vi "WriteScript.vi"() -> ()   [LabVIEW 2015]
uses:
  <vilib>/Utility/file.llb/Write Delimited Spreadsheet (string).vi
  Users/Sherman/Desktop/BETA_GSCS/GUI/GSP_GUI_global.vi
  <vilib>/Utility/file.llb/Read Delimited Spreadsheet (string).vi
panel:
  out "Expected Runtime":dbl
  in  "Script":string[](array[string])
  out "Gratings":T1(array[cluster])
  out "Array":T2(array[cluster])
  in  "Master Config Location":path
  in  "Littrow Config":dbl
  in  "focus sequence":bool
  in  "Clear line":bool
  out "(s)":dbl caption="Expected Runtime"
  in  "Save":bool
  in  "Line Number":dbl=1.0 min=0.0 step=1.0
  in  "Open script":bool
  in  "text file":refnum<file>
  in  "Script Name":string
  out "status":string
  in  "Add to Script Button":bool
  in  "Location of Script File":path=path "C:/GSCS Scripting/Scripts"
  in  "cluster":T3={"SI camera info"={"Observer Name"="", "object name"="", "File name base"="", "Camera Color"="Red", "Exp type tab"="", "Number of Exp"=1, "Exp time"=0.0, "CCD Readout Speed"=5, "CCD ROI Mode"=10, "Hg(Ar)"=FALSE, "Cu"=FALSE, "Ne"=FALSE, "Bulb"=FALSE, "Ar"=FALSE, "Quartz"=FALSE, "Quartz Percent"=0, "Fe"=FALSE, "Notes"="", "Target Number"="", "DomePercent"=0, "Dome"=FALSE, "Start"=0.0, "Delta"=0.0, "Steps"=0.0, "Custom Roi"={0, 4096, 1, 0, 4096, 1}}, "Configuration"={"Primary Filter"="<NO FILTER>", "Secondary Filter"="<NO FILTER>", "Slit Mask"="<NO MASK>", "Grating"="<NO GRATING>", "CS Target"=0.0, "GS Target"=0.0, "Coll Focus"=1000, "Camera Focus"=0, "Name"="", "User"="", "Date"="", "Comment"="", "use Flexure Comp?"=TRUE, "Select Mode:"=0}, "RA (HH:MM:SS.SS)"="-00:00:00.00", "DEC (HH:MM:SS.SS)"="-00:00:00.00"} {"Configuration"."Select Mode:" items=["Custom", "Imaging", "300 All", "600 UV", "600 Blue", "600 Mid", "600 Red", "1200 m0", "1200 m1", "1200 m2", "1200 m3", "1200 m4", "1200 m5", "1200 m6", "1200 m7", "1200 RESOLVE", "400 m1", "400 m2", "930 m1", "930 m2", "930 m3", "930 m4", "930 m5", "930 m6", "400WD", "930TP", "400Fermi", "400Padgett", "400Lewis", "400Crotts", "600BLee", "600RLee", "400WW", "ZZ Ceti Red", "ZZ Ceti Blue"]; "SI camera info"."DomePercent" min=0 step=1; "SI camera info"."Quartz Percent" min=0 step=1; "SI camera info"."CCD Readout Speed" items=["50 kHz, ATTN 0", "50 kHz, ATTN 2", "50 kHz, ATTN 3", "100 kHz, ATTN 0", "100 kHz, ATTN 2", "100 kHz, ATTN 3", "200 kHz, ATTN 0", "200 kHz, ATTN 2", "400 kHz, ATTN 0"]; "SI camera info"."CCD ROI Mode" items=["Imaging, 1x1  "=0, "Imaging, 2x2"=1, "Imaging, 3x3"=2, "Spectroscopic, 1x1"=3, "Spectroscopic, 2x2"=4, "Spectroscopic, 3x3"=5, "MOS, 1x1"=11, "MOS, 2x2"=12, "MOS, 3x3"=13, "Slicer"=6, "Spectroscopic, ZZ Ceti"=14, "Slit Imaging/Alignment"=7, "MOS Imaging/Alignment"=10, "Set user-defined ROI..."=21, "Custom Mode"=9]; "SI camera info"."Number of Exp" min=0 step=1; "SI camera info"."Exp time" min=0.0 format="%#.1f"}
  # "Central Wavelength (mm)"
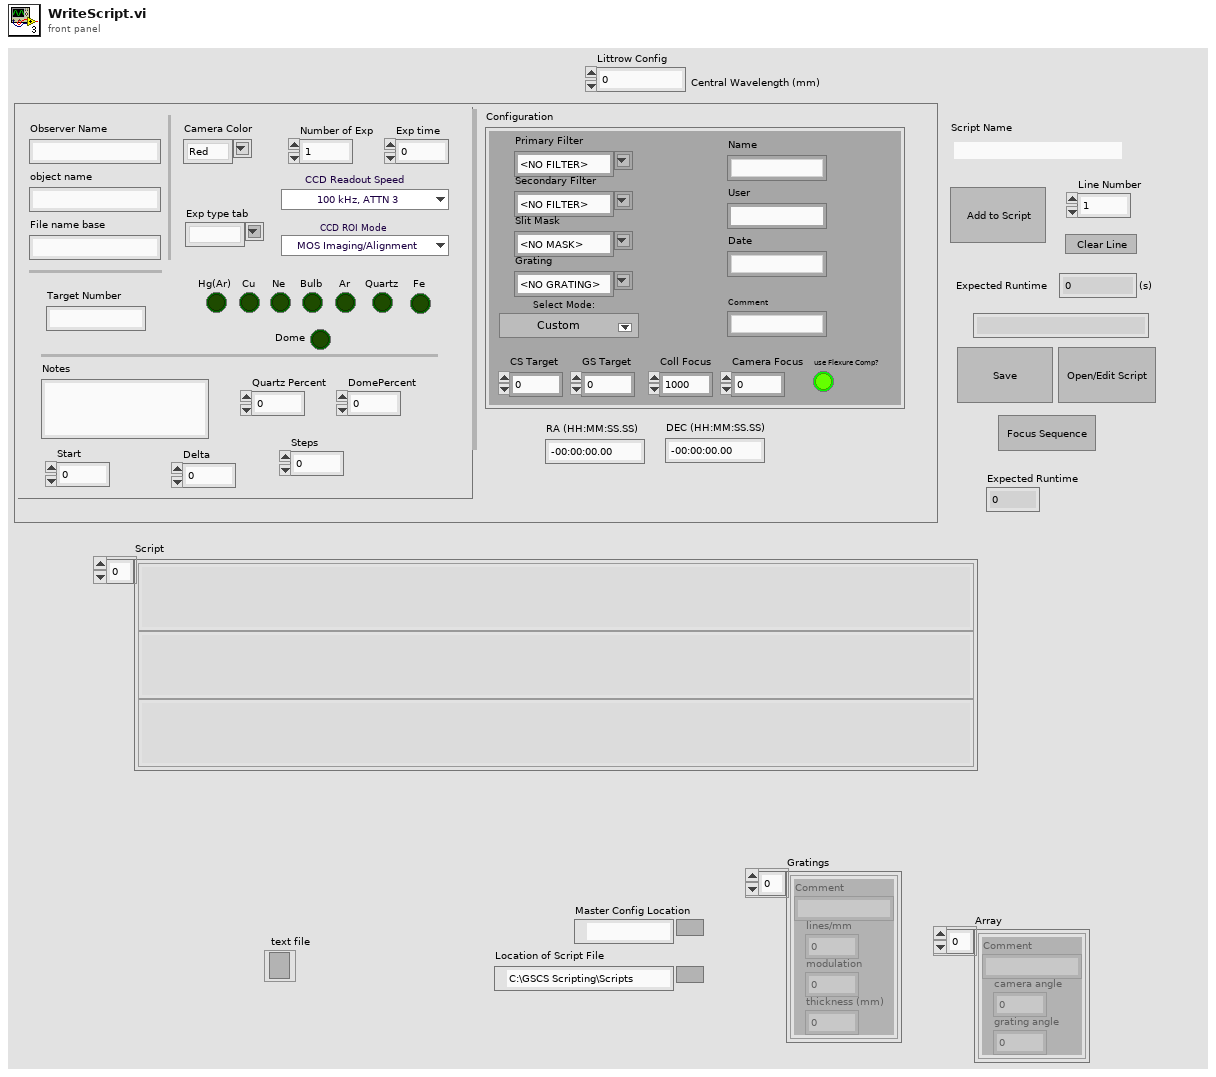
[diagram p1: front panel]
types:
  T1 = cluster{"Comment":string, "lines/mm":i32, "modulation":dbl, "thickness (mm)":dbl}[]
  T2 = cluster{"Comment":string, "camera angle":dbl, "grating angle":dbl}[]
  T3 = cluster{"SI camera info":cluster{"Observer Name":string, "object name":string, "File name base":string, "Camera Color":string, "Exp type tab":string, "Number of Exp":i32, "Exp time":dbl, "CCD Readout Speed":u8, "CCD ROI Mode":u16, "Hg(Ar)":bool, "Cu":bool, "Ne":bool, "Bulb":bool, "Ar":bool, "Quartz":bool, "Quartz Percent":i32, "Fe":bool, "Notes":string, "Target Number":string, "DomePercent":i32, "Dome":bool, "Start":dbl, "Delta":dbl, "Steps":dbl, "Custom Roi":cluster{i32, i32, i32, i32, i32, i32}}, "Configuration":cluster{"Primary Filter":string, "Secondary Filter":string, "Slit Mask":string, "Grating":string, "CS Target":dbl, "GS Target":dbl, "Coll Focus":i32, "Camera Focus":i32, "Name":string, "User":string, "Date":string, "Comment":string, "use Flexure Comp?":bool, "Select Mode:":u16}, "RA (HH:MM:SS.SS)":string, "DEC (HH:MM:SS.SS)":string}
  T4 = cluster{"Comment":string, "lines/mm":i32, "modulation":dbl, "thickness (mm)":dbl}
  T5 = cluster{"Serial Origin":i32, "Serial Length":i32, "Serial Binning":i32, "Parallel Origin":i32, "Parallel Length":i32, "Parallel Binning":i32}
  T6 = cluster{"Primary Filter Names":string[], "Secondary Filter Names":string[], "Grating Names":string[], "Slit Mask Names":string[], "Standard Observing Modes":string[]}
  T7 = cluster{"Comment":string, "camera angle":dbl, "grating angle":dbl}
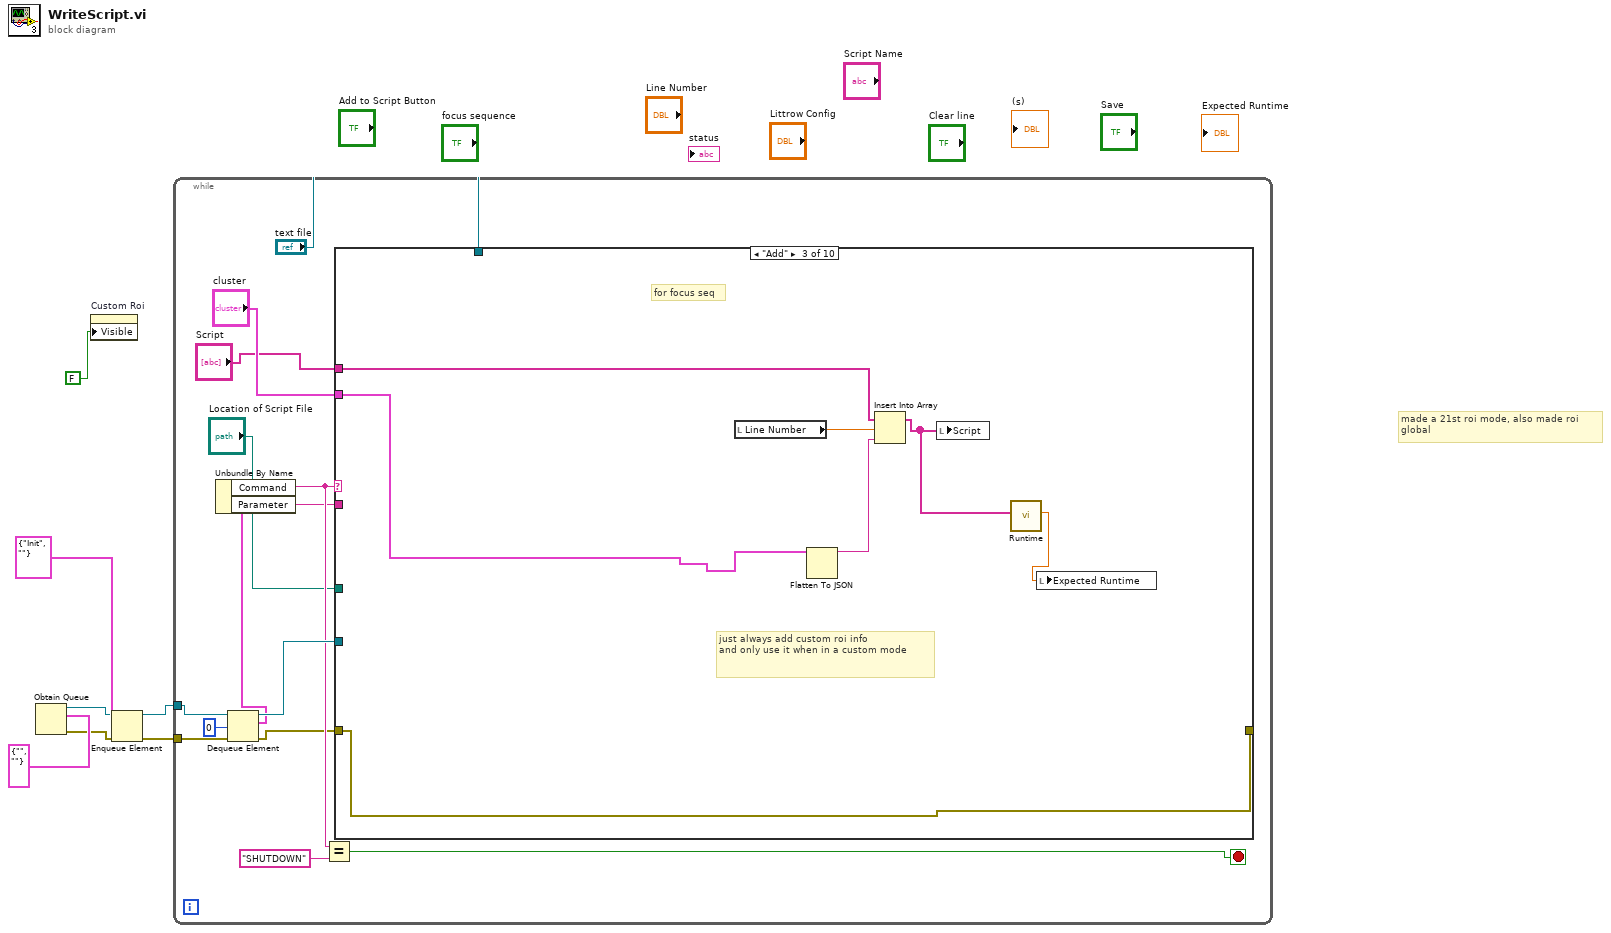
[diagram p0: block diagram]
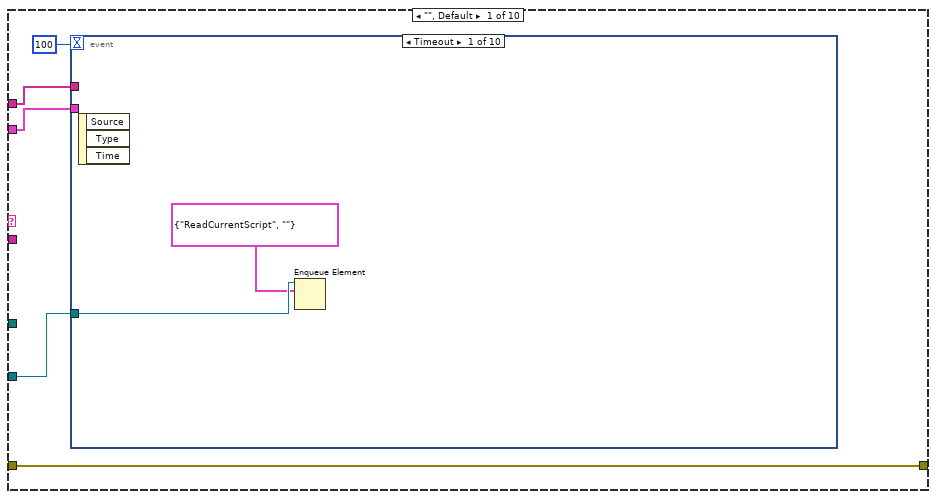
[diagram p2: hidden frame]
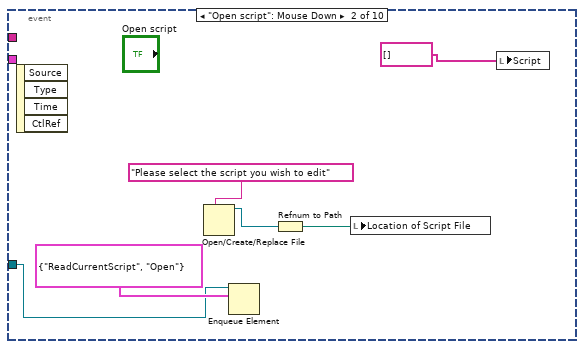
[diagram p3: hidden frame]
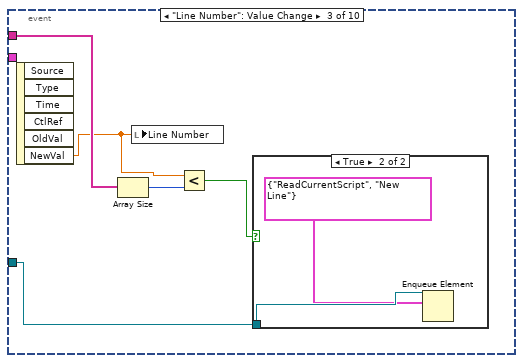
[diagram p4: hidden frame]
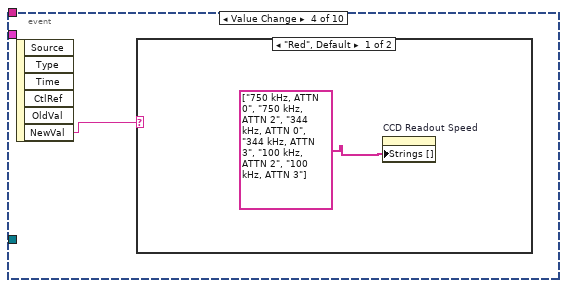
[diagram p6: hidden frame]
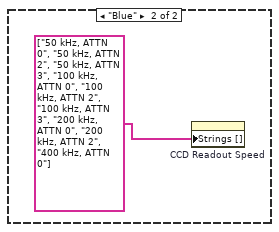
[diagram p7: hidden frame]
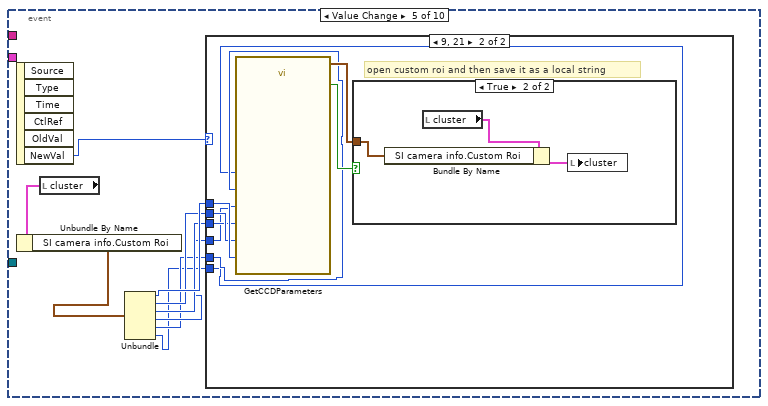
[diagram p8: hidden frame]
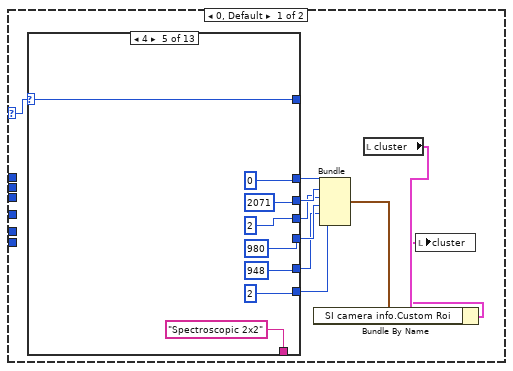
[diagram p9: hidden frame]
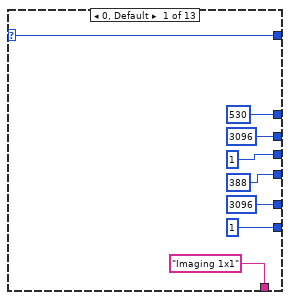
[diagram p10: hidden frame]
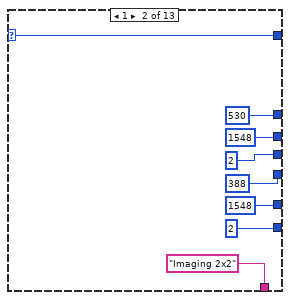
[diagram p11: hidden frame]
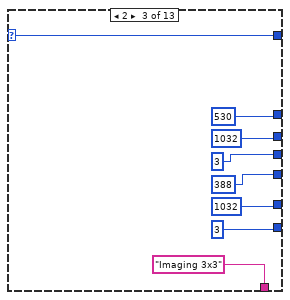
[diagram p12: hidden frame]
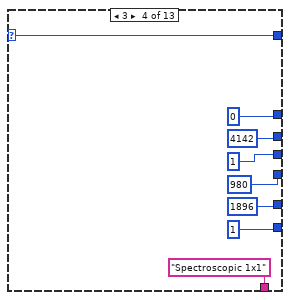
[diagram p13: hidden frame]
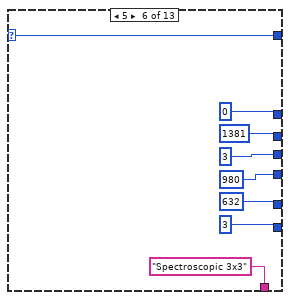
[diagram p14: hidden frame]
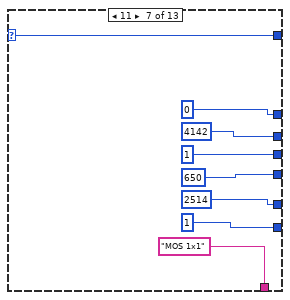
[diagram p15: hidden frame]
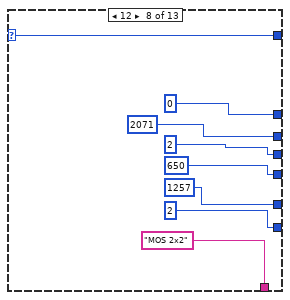
[diagram p16: hidden frame]
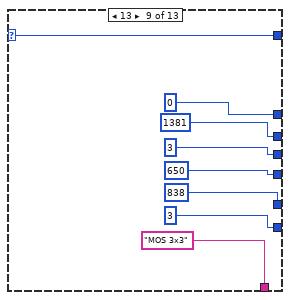
[diagram p17: hidden frame]
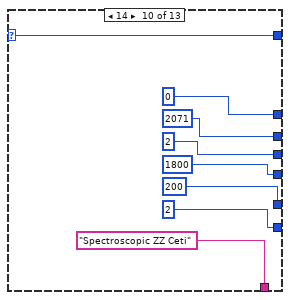
[diagram p18: hidden frame]
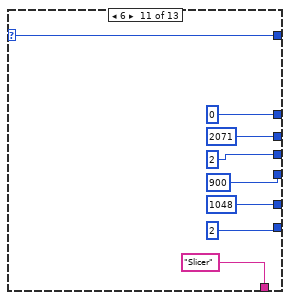
[diagram p19: hidden frame]
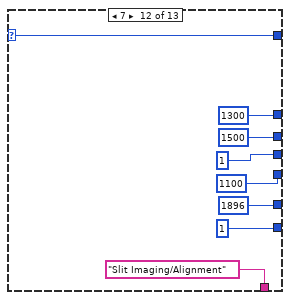
[diagram p20: hidden frame]
diagram:
  # "made a 21st roi mode, also made roi\nglobal"
  n1 = Obtain Queue(element data type=cluster{"\nCommand":string, "Parameter":string} {"\nCommand"="", "Parameter"=""}) -> (queue out=w5:refnum<queue>, error out=w3:errorcluster)  [unwired: 4 in, 1 out]
  n2 = property on="Custom Roi" class="Clust (strict)"("Visible"=FALSE) -> ()  [unwired: 2 in, 2 out]
  n3 = Enqueue Element(queue=w5, element=cluster{string, string} {"Init", ""}, error in (no error)=w3) -> (queue out=w4:refnum<queue>, error out=w2:errorcluster)  [unwired: 1 in, 1 out]
  n4 = while {
    tunnel: w4 -> [w13]
    tunnel: w2 -> [w12]
    stop <- w17 stop-if-true
    n5 = Dequeue Element(queue=w13, timeout in ms (-1)=0, error in (no error)=w12) -> (queue out=w21:refnum<queue>, element=w20:cluster{"\nCommand":string, "Parameter":string}, error out=w11:errorcluster)  [unwired: 1 out]
    n6 = Unbundle By Name(w20) -> ("Command"=w18:string, "Parameter"=w16:string)
    n7 = Equal?(x=w18, y="SHUTDOWN") -> (x = y?=w17:bool)
    n8 = case shown="\"Add\"" w18 {
      tunnel: w21 -> [w26 w220 _ _ _ w247 _ _ _ _]
      tunnel: w16 -> [_ _ _ _ _ _ _ _ _ w314]
      tunnel: "cluster" -> [w22 w213 w225 _ w238 _ _ _ _ _]
      tunnel: "Location of Script File" -> [_ _ _ w235 _ _ _ _ _ w317]
      tunnel: w11 -> [w25 w221 w228 w234 w242 w253 w255 w270 w299 w316]
      tunnel: [w25 w221 w228 w233 w242 w253 w254 w269 w298 w315] -> _
      tunnel: "text file" -> [_ _ _ _ _ _ _ _ _ _]
      tunnel: "Script" -> [w23 _ w224 w230 _ _ _ _ _ w313]
      frame "", Default {
        n9 = event shown="[0] Timeout" {
          selector: _ -> [_ _ _ _ _ _ _ _ _ _]
          dyn-events: _ -> [_ _ _ _ _ _ _ _ _ _]
          timeout: 100 -> [_ _ _ _ _ _ _ _ _ _]
          tunnel: w26 -> [w28 w30 w39 _ _ w184 w196 _ w201 _]
          tunnel: w23 -> [_ _ w38 _ _ _ w194 w200 _ _]
          tunnel: w22 -> [_ _ _ _ _ w183 _ _ _ _]
          event Timeout {
            n10 = event-data() -> ()  [unwired: 1 in, 3 out]
            n11 = Enqueue Element(queue=w28, element=cluster{string, string} {"ReadCurrentScript", ""}) -> ()  [unwired: 2 in, 3 out]
          }
          event "Open script": Mouse Down {
            n12 = event-data() -> ()  [unwired: 1 in, 4 out]
            n13 = Open/Create/Replace File(prompt="Please select the script you wish to edit") -> (refnum out=w33:refnum<file>)  [unwired: 5 in, 2 out]
            n14 = Enqueue Element(queue=w30, element=cluster{string, string} {"ReadCurrentScript", "Open"}) -> ()  [unwired: 2 in, 3 out]
            n15 = Refnum to Path(1:w33) -> (0:w32:path)
            n16 = local write "Location of Script File"(w32) -> ()
            n17 = local write "Script"(string[] []) -> ()
          }
          event "Line Number": Value Change {
            n18 = event-data() -> ("NewVal"=w37:dbl)  [unwired: 1 in, 5 out]
            n19 = Array Size(array=w38) -> (size(s)=w35:i32)
            n20 = local write "Line Number"(w37) -> ()
            n21 = Less?(x=w37, y=w35) -> (x < y?=w36:bool)
            n22 = case shown="True" w36 {
              tunnel: w39 -> [_ w41]
              frame False {
              }
              frame True {
                n23 = Enqueue Element(queue=w41, element=cluster{string, string} {"ReadCurrentScript", "New Line"}) -> ()  [unwired: 2 in, 3 out]
              }
            }
          }
          event "cluster.SI camera info.Camera Color": Value Change {
            n24 = event-data() -> ("NewVal"=w42:string)  [unwired: 1 in, 5 out]
            n25 = case shown="\"Red\", Default" w42 {
              frame "Red", Default {
                n26 = property on="CCD Readout Speed" class="Ring (strict)"("Strings []"=string[] ["750 kHz, ATTN 0", "750 kHz, ATTN 2", "344 kHz, ATTN 0", "344 kHz, ATTN 3", "100 kHz, ATTN 2", "100 kHz, ATTN 3"]) -> ()  [unwired: 2 in, 2 out]
              }
              frame "Blue" {
                n27 = property on="CCD Readout Speed" class="Ring (strict)"("Strings []"=string[] ["50 kHz, ATTN 0", "50 kHz, ATTN 2", "50 kHz, ATTN 3", "100 kHz, ATTN 0", "100 kHz, ATTN 2", "100 kHz, ATTN 3", "200 kHz, ATTN 0", "200 kHz, ATTN 2", "400 kHz, ATTN 0"]) -> ()  [unwired: 2 in, 2 out]
              }
            }
          }
          event "cluster.SI camera info.CCD ROI Mode": Value Change {
            n28 = event-data() -> ("NewVal"=w53:u16)  [unwired: 1 in, 5 out]
            n29 = local read "cluster"() -> (w52:T3)
            n30 = Unbundle By Name(w52) -> ("SI camera info.Custom Roi"=w51:cluster{i32, i32, i32, i32, i32, i32})
            n31 = Unbundle(w51) -> (w50:i32, w49:i32, w48:i32, w47:i32, w46:i32, w45:i32)
            n32 = case shown="9, 21" w53 {
              selector: w53 -> [w63 _]
              tunnel: w50 -> [_ w173]
              tunnel: w49 -> [_ w172]
              tunnel: w48 -> [_ w171]
              tunnel: w47 -> [_ w170]
              tunnel: w46 -> [_ w169]
              tunnel: w45 -> [_ w168]
              frame 0, Default {
                n33 = case shown="4" w63 {
                  selector: w63 -> [w64 w72 w80 w88 w96 w104 w112 w120 w128 w136 w151 w152 w160]
                  tunnel: [530 530 530 0 0 0 0 0 0 0 0 1300 1300] -> w62
                  tunnel: [3096 1548 1032 4142 2071 1381 4142 2071 1381 2071 2071 1500 1500] -> w61
                  tunnel: [1 2 3 1 2 3 1 2 3 2 2 1 1] -> w60
                  tunnel: [388 388 388 980 980 980 650 650 650 1800 900 1100 790] -> w59
                  tunnel: [3096 1548 1032 1896 948 632 2514 1257 838 200 1048 1896 2370] -> w58
                  tunnel: [1 2 3 1 2 3 1 2 3 2 2 1 1] -> w57
                  tunnel: ["Imaging 1x1" ("Current Status") "Imaging 2x2" ("Current Status") "Imaging 3x3" ("Current Status") "Spectroscopic 1x1" ("Current Status") "Spectroscopic 2x2" ("Current Status") "Spectroscopic 3x3" ("Current Status") "MOS 1x1" ("Current Status") "MOS 2x2" ("Current Status") "MOS 3x3" ("Current Status") "Spectroscopic ZZ Ceti" ("Current Status") "Slicer" ("Current Status") "Slit Imaging/Alignment" ("Current Status") "MOS Imaging/Alignment" ("Current Status")] -> _
                  tunnel: [w64 w72 w80 w88 w96 w104 w112 w120 w128 w136 w151 w152 w160] -> _
                  frame 0, Default {
                  }
                  frame 1 {
                  }
                  frame 2 {
                  }
                  frame 3 {
                  }
                  frame 4 {
                  }
                  frame 5 {
                  }
                  frame 11 {
                  }
                  frame 12 {
                  }
                  frame 13 {
                  }
                  frame 14 {
                  }
                  frame 6 {
                  }
                  frame 7 {
                  }
                  frame 10 {
                  }
                }
                n34 = Bundle(w62, w61, w60, w59, w58, w57) -> (w55:cluster{i32, i32, i32, i32, i32, i32})  [unwired: 1 in]
                n35 = local read "cluster"() -> (w56:T3)
                n36 = Bundle By Name(cluster=w56, "SI camera info.Custom Roi"=w55) -> (w54:T3)
                n37 = local write "cluster"(w54) -> ()
              }
              frame 9, 21 {
                # "open custom roi and then save it as a local string"
                n38 = call "GetCCDParameters.vi"("Serial Origin"=w173, "Parallel Origin"=w170, "Serial Length"=w172, "Parallel Length"=w169, "Serial Binning"=w171, "Parallel Binning"=w168) -> ("CCD Format Parameters"=w175:T5, "Set Parameters"=w174:bool)  [unwired: 10 in, 2 out]
                n39 = case shown="True" w174 {
                  tunnel: w175 -> [_ w176]
                  frame False {
                  }
                  frame True {
                    n40 = local read "cluster"() -> (w178:T3)
                    n41 = Bundle By Name(cluster=w178, "SI camera info.Custom Roi"=w176) -> (w177:T3)
                    n42 = local write "cluster"(w177) -> ()
                  }
                }
              }
            }
          }
          event "focus sequence": Value Change {
            n43 = event-data() -> ("NewVal"=w186:bool)  [unwired: 1 in, 5 out]
            n44 = call "Focus Sequence"("Enable"=w186) -> ("Number of steps"=w180:dbl, "Delta"=w181:dbl, "Starting focus value"=w182:dbl, "Done"=w185:bool)  [unwired: 14 in, 1 out]
            n45 = Bundle By Name(cluster=w183, "SI camera info.Start"=w182, "SI camera info.Delta"=w181, "SI camera info.Steps"=w180) -> (w179:T3)
            n46 = case shown="True" w185 {
              tunnel: w184 -> [_ w187]
              frame False {
              }
              frame True {
                n47 = Enqueue Element(queue=w187, element=cluster{string, string} {"Focus_Sequence", ""}) -> ()  [unwired: 2 in, 3 out]
              }
            }
            n48 = local write "cluster"(w179) -> ()
          }
          event "Add to Script Button": Mouse Up {
            n49 = event-data() -> ()  [unwired: 1 in, 8 out]
            n50 = local read "Line Number"() -> (w195:dbl)
            n51 = Array Size(array=w194) -> (size(s)=w189:i32)
            n52 = Greater?(x=w195, y=w189) -> (0:w193:bool)
            n53 = case shown="False" w193 {
              tunnel: w189 -> [_ w197]
              frame False {
              }
              frame True {
                n54 = local write "Line Number"(w197) -> ()
              }
            }
            n55 = Enqueue Element(queue=w196, element=cluster{string, string} {"Add", ""}) -> (queue out=w190:refnum<queue>)  [unwired: 2 in, 2 out]
            n56 = Enqueue Element(queue=w190, element=cluster{string, string} {"PostAdd", ""}) -> ()  [unwired: 2 in, 3 out]
          }
          event "Clear line": Value Change {
            n57 = event-data() -> ()  [unwired: 1 in, 6 out]
            n58 = local read "Line Number"() -> (w198:dbl)
            n59 = Delete From Array(array=w200, index=w198) -> (array with subset deleted=w199:string[])  [unwired: 1 in, 1 out]
            n60 = local write "Script"(w199) -> ()
          }
          event "Save": Mouse Down {
            n61 = event-data() -> ()  [unwired: 1 in, 8 out]
            n62 = Enqueue Element(queue=w201, element=cluster{string, string} {"Save", ""}) -> ()  [unwired: 2 in, 3 out]
          }
          event "Script Name": Value Change {
            n63 = event-data() -> ()  [unwired: 1 in, 6 out]
            n64 = local read "Script Name"() -> (w203:string)
            n65 = Current VI's Path() -> (path=w210:path)
            n66 = Strip Path(path=w210) -> (stripped path=w209:path)  [unwired: 1 out]
            n67 = Build Path(base path=w209, name or relative path="Scripts") -> (appended path=w205:path)
            n68 = Concatenate Strings(w203, ".txt") -> (w206:string)
            n69 = Build Path(base path=w205, name or relative path=w206) -> (appended path=w204:path)
            n70 = local write "Location of Script File"(w204) -> ()
          }
        }
      }
      frame "Focus_Sequence" {
        n71 = Bundle By Name(cluster=w213, "SI camera info.Exp type tab"="Focus") -> (w212:T3)
        n72 = local write "cluster"(w212) -> ()
        n73 = Bundle("Add", "") -> (w215:cluster{string, string})  [unwired: 1 in]
        n74 = Enqueue Element(queue=w220, element=w215) -> (queue out=w218:refnum<queue>, error out=w217:errorcluster)  [unwired: 2 in, 1 out]
        n75 = Enqueue Element(queue=w218, element=cluster{string, string} {"PostAdd", ""}, error in (no error)=w217) -> ()  [unwired: 1 in, 3 out]
      }
      frame "Add" {
        # "for focus seq"
        # "just always add custom roi info\nand only use it when in a custom mode"
        n76 = local read "Line Number"() -> (w226:dbl)
        n77 = Flatten To JSON(anything=w225) -> (JSON string=w227:string)  [unwired: 2 in, 1 out]
        n78 = Insert Into Array(array=w224, index=w226, new element=w227) -> (w223:string[])
        n79 = local write "Script"(w223) -> ()
        n80 = call "Runtime.vi"("Script"=w223) -> ("Runtime"=w222:dbl)  [unwired: 10 in]
        n81 = local write "Expected Runtime"(w222) -> ()
      }
      frame "Save" {
        n82 = call-poly <vilib>:"Write Delimited Spreadsheet.vi"("file path (dialog if empty)"=w235, "1D data"=w230, "append to file? (F)"=FALSE, "error in (no error)"=w234, "delimiter (\\t)"="\r") -> ("error out"=w233:errorcluster)  [unwired: 9 in, 1 out]
        n83 = local write "status"("Script Saved!") -> ()
      }
      frame "PostAdd" {
        w237 = 0.0
        n84 = Bundle By Name(cluster=w238, "SI camera info.Start"=w237, "SI camera info.Delta"=w237, "SI camera info.Steps"=w237) -> (w236:T3)
        n85 = local write "cluster"(w236) -> ()
        n86 = local read "Line Number"() -> (w239:dbl)
        n87 = local write "status"("Line added to Script!") -> ()
        n88 = Increment(x=w239) -> (x+1=w240:dbl)
        n89 = local write "Line Number"(w240) -> ()
      }
      frame "Init" {
        n90 = Enqueue Element(queue=w247, element=cluster{string, string} {"Init Config", ""}) -> (queue out=w244:refnum<queue>)  [unwired: 2 in, 2 out]
        n91 = Enqueue Element(queue=w244, element=cluster{string, string} {"Read Config Info", ""}) -> (queue out=w243:refnum<queue>)  [unwired: 2 in, 2 out]
        n92 = local write "Script"(string[] []) -> ()
        n93 = local write "Line Number"(1.0) -> ()
        n94 = Enqueue Element(queue=w243, element=cluster{string, string} {"Read Grating Info", ""}) -> ()  [unwired: 2 in, 3 out]
        n95 = property on="Script Name" class="Str"("Value"="") -> ()  [unwired: 2 in, 2 out]
        n96 = local write "(s)"(0) -> ()
      }
      frame "Init Config" {
        # "only gets the number\nof slots for each"
        n97 = Two Button Dialog(message="To determine which setups are availbe, please provide information about your mastr configuration file.", 1:"Use new (select path)", 2:"Use current") -> (T button?=w260:bool)
        n98 = case shown="True" w260 {
          tunnel: ["Master Config Location" path "\\\\SHERMAN-PC\\Config/masterconfig.ini"] -> w256
          frame False {
          }
          frame True {
          }
        }
        n99 = call "Read_Master_Config.vi"("error in (no error)"=w255, "configuration file path"=w256) -> ("error out"=w254:errorcluster, "Present Configuration"=w262:T6)  [unwired: 3 in, 1 out]
        n100 = Unbundle By Name(w262) -> ("Primary Filter Names"=w263:string[], "Secondary Filter Names"=w264:string[], "Grating Names"=w265:string[], "Slit Mask Names"=w266:string[], "Standard Observing Modes"=w261:string[])
        n101 = global write "GSP_GUI_global.vi" "Standard Observing Mode Names"(w261) -> ()
        n102 = global write "GSP_GUI_global.vi" "Primary Filter Names"(w263) -> ()
        n103 = global write "GSP_GUI_global.vi" "Secondary Filter Names"(w264) -> ()
        n104 = global write "GSP_GUI_global.vi" "Slit Mask Names"(w266) -> ()
        n105 = global write "GSP_GUI_global.vi" "Grating Names"(w265) -> ()
      }
      frame "Read Config Info" {
        n106 = global read "GSP_GUI_global.vi" "Primary Filter Names"() -> (w287:string[])
        n107 = global read "GSP_GUI_global.vi" "Secondary Filter Names"() -> (w275:string[])
        n108 = global read "GSP_GUI_global.vi" "Slit Mask Names"() -> (w281:string[])
        n109 = global read "GSP_GUI_global.vi" "Standard Observing Mode Names"() -> (w272:string[])
        n110 = Insert Into Array(array=w287, index=0, new element="<NO FILTER>" ("new element/subarray")) -> (w285:string[])
        n111 = Insert Into Array(array=w281, index=0, new element="<NO MASK>" ("new element/subarray")) -> (w278:string[])
        n112 = Insert Into Array(array=w275, index=0, new element="<NO FILTER>" ("new element/subarray")) -> (w274:string[])
        n113 = property on="Slit Mask" class="CmbBox"("Strings[]"=w278) -> ()  [unwired: 2 in, 2 out]
        n114 = Index Array(array=w285, index=5) -> (element=w283:string)
        n115 = property on="Secondary Filter" class="CmbBox"("Strings[]"=w274) -> ()  [unwired: 2 in, 2 out]
        n116 = property on="Select Mode:" class="Ring (strict)"("Strings []"=w272) -> ()  [unwired: 2 in, 2 out]
        n117 = case shown="\"SQUARE\"" w283 {
          tunnel: w285 -> [w294 w297]
          tunnel: [w294 w295] -> w282
          frame "", Default {
            (unwired) FALSE ("5 hole or 6 hole wheel?")
          }
          frame "SQUARE" {
            n118 = Delete From Array(array=w297, index=5) -> (array with subset deleted=w295:string[])  [unwired: 1 in, 1 out]
          }
        }
        n119 = for {
          tunnel: w272 -> [w292] mode=indexing
          tunnel: path "\\\\SHERMAN-PC\\Config/observing_modes.ini" -> [w293]
          tunnel: w270 -> [w291]
          tunnel: [w290] -> w269
          tunnel: [w289] -> w273 mode=indexing
          n120 = call "get_std_observing_modes.vi"("error in (no error)"=w291, "mode name"=w292, "configuration file path"=w293) -> ("error out"=w290:errorcluster, "Standard Mode Info"=w289:T7)  [unwired: 3 in]
        }
        "Array" <- w273
        n121 = property on="Primary Filter" class="CmbBox"("Strings[]"=w282) -> ()  [unwired: 2 in, 2 out]
      }
      frame "Read Grating Info" {
        n122 = global read "GSP_GUI_global.vi" "Grating File"() -> (w304:path)
        n123 = global read "GSP_GUI_global.vi" "Grating Names"() -> (w300:string[])
        n124 = for {
          tunnel: [w312] -> w303 mode=indexing
          tunnel: [w311] -> w298
          tunnel: w300 -> [w310] mode=indexing
          tunnel: w304 -> [w309]
          tunnel: w299 -> [w308]
          n125 = call "get_grating_info.vi"("error in (no error)"=w308, "grating name"=w310, "configuration file path"=w309) -> ("error out"=w311:errorcluster, "Grating Info"=w312:T4)  [unwired: 3 in]
        }
        n126 = Build Array (concatenate)(T4 {"Comment"="", "lines/mm"=0, "modulation"=0.0, "thickness (mm)"=0.0} ("Grating Info"), w303) -> (→"Gratings":T1)
        n127 = Insert Into Array(array=w300, index=0, new element="<NO GRATING>" ("new element/subarray")) -> (w305:string[])
        n128 = property on="Grating" class="CmbBox"("Strings[]"=w305) -> ()  [unwired: 2 in, 2 out]
      }
      frame "ReadCurrentScript" {
        n129 = case shown="\"Open\"" w314 {
          tunnel: w317 -> [_ w324 _]
          tunnel: w316 -> [w318 w334 w340]
          tunnel: [w318 w333 w340] -> w315
          tunnel: w313 -> [_ _ w341]
          frame "", Default {
          }
          frame "Open" {
            n130 = call-poly <vilib>:"Read Delimited Spreadsheet.vi"("file path (dialog if empty)"=w324, "number of rows (all:-1)"=-1, "error in (no error)"=w334, "delimiter (\\t)"="\r") -> ("all rows"=w327:string[][], "error out"=w333:errorcluster)  [unwired: 6 in, 4 out]
            n131 = local read "Line Number"() -> (w330:dbl)
            n132 = local read "cluster"() -> (w332:T3)
            n133 = Index Array(array=w327, index (col)=0) -> (element=w326:string[])  [unwired: 1 in]
            n134 = Index Array(array=w326, index=w330) -> (element=w329:string)
            n135 = Unflatten From JSON(JSON string=w329, type and defaults=w332) -> (value=w331:T3)  [unwired: 5 in, 1 out]
            n136 = local write "Script"(w326) -> ()
            n137 = local write "cluster"(w331) -> ()
            n138 = Strip Path(path=w324) -> (name=w322:string)  [unwired: 1 out]
            n139 = String Length(string=w322) -> (length=w321:i32)
            n140 = Subtract(x=w321, y=4) -> (x-y=w320:i32)
            n141 = String Subset(string=w322, length (rest)=w320) -> (substring=w323:string)  [unwired: 1 in]
            n142 = local write "Script Name"(w323) -> ()
          }
          frame "New Line" {
            n143 = local read "Line Number"() -> (w339:dbl)
            n144 = local read "cluster"() -> (w336:T3)
            n145 = Index Array(array=w341, index=w339) -> (element=w338:string)
            n146 = Unflatten From JSON(JSON string=w338, type and defaults=w336) -> (value=w337:T3)  [unwired: 5 in, 1 out]
            n147 = local write "cluster"(w337) -> ()
          }
        }
      }
    }
  }
